vi "4200_strings.vi"() -> ()   [LabVIEW 2013]
panel:
  in  "number 3":dbl
  in  "number 2":dbl
  in  "Number of points":dbl
  in  "SMU2 Output":T1(ring)
  in  "SMU2 Function":enum16{"Sweep", "Step", "Constant"}(ring)
  in  "SMU1 Function":enum16{"Sweep", "Step", "Constant"}(ring)
  in  "SMU1 Output":T1(ring)
  # "SMU2"
  # "SMU1"
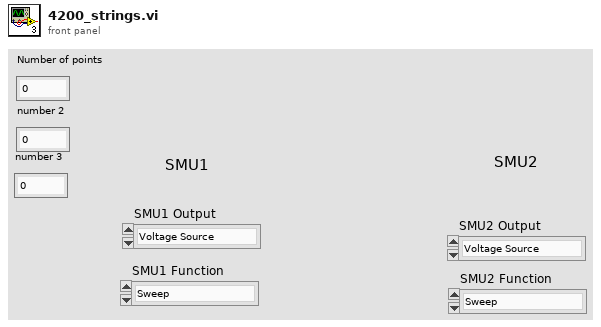
[diagram p1: front panel]
types:
  T1 = enum16{"Voltage Source", "Current Source", "COM"}
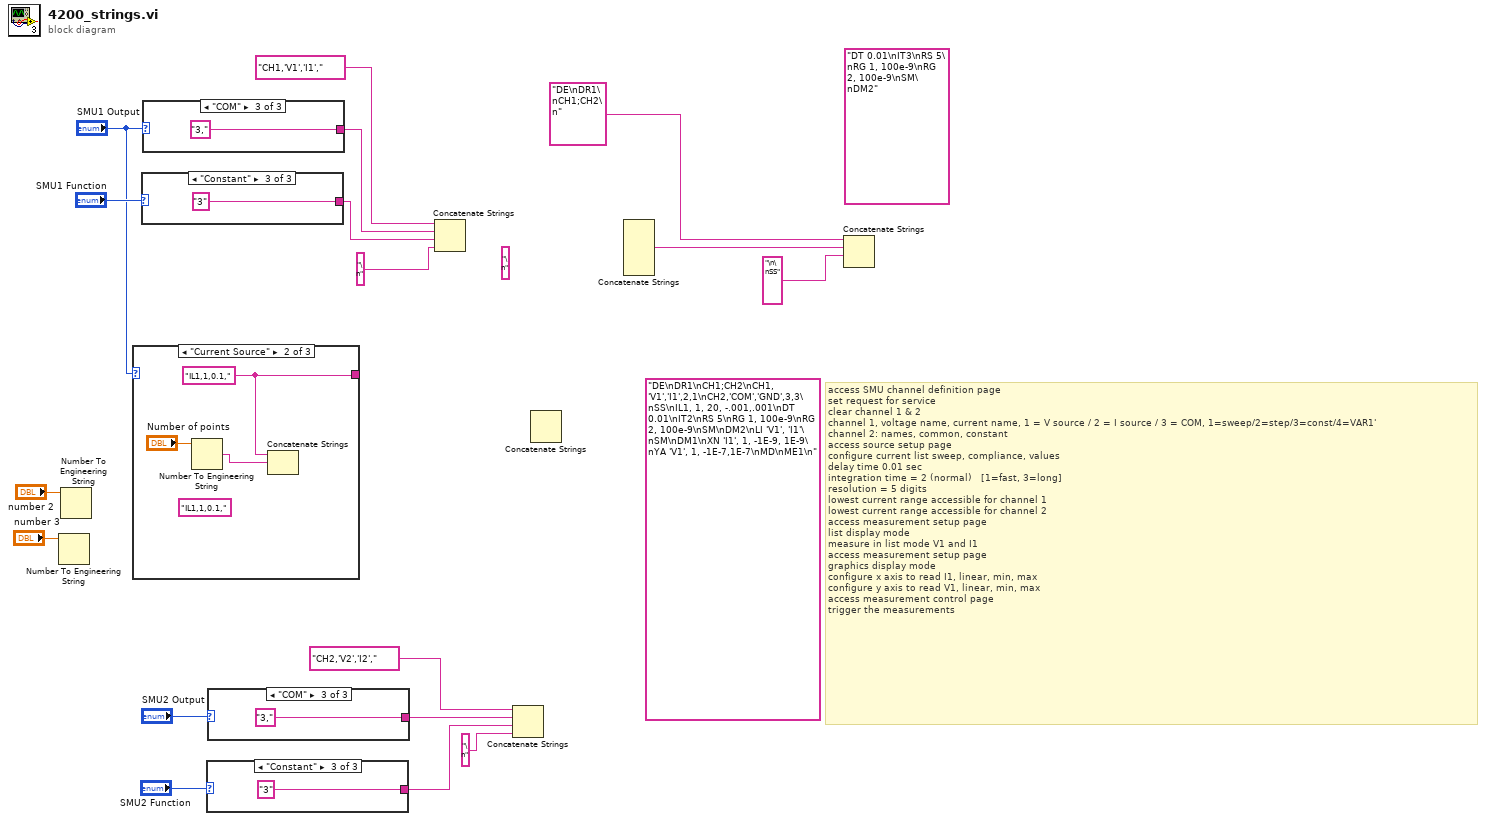
[diagram p0: block diagram]
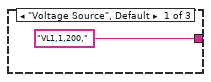
[diagram p2: hidden frame]
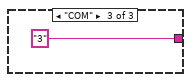
[diagram p3: hidden frame]
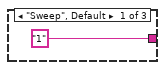
[diagram p4: hidden frame]
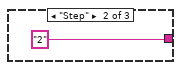
[diagram p5: hidden frame]
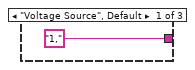
[diagram p6: hidden frame]
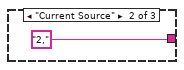
[diagram p7: hidden frame]
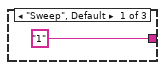
[diagram p8: hidden frame]
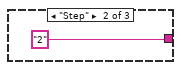
[diagram p9: hidden frame]
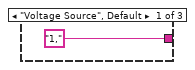
[diagram p10: hidden frame]
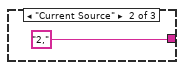
[diagram p11: hidden frame]
diagram:
  (unwired) "DE\nDR1\nCH1;CH2\nCH1, 'V1','I1',2,1\nCH2,'COM','GND',3,3\nSS\nIL1, 1, 20, -.001,.001\nDT 0.01\nIT2\nRS 5\nRG 1, 100e-9\nRG 2, 100e-9\nSM\nDM2\nLI 'V1', 'I1'\nSM\nDM1\nXN 'I1', 1, -1E-9, 1E-9\nYA 'V1', 1, -1E-7,1E-7\nMD\nME1\n" ("write buffer")
  (unwired) "DT 0.01\nIT3\nRS 5\nRG 1, 100e-9\nRG 2, 100e-9\nSM\nDM2" ("string")
  (unwired) "\n" ("string")
  # "access SMU channel definition page\nset request for service\nclear channel 1 & 2\nchannel 1, voltage name, current name, 1 = V source / 2 = I source / 3 = COM, 1=sweep/2=step/3=const/4=VAR1' \nchannel 2: names, common, constant\naccess source setup page\nconfigure current list sweep, compliance, values\ndelay time 0.01 sec\nintegration time = 2 (normal)   [1=fast, 3=long]\nresolution = 5 digits\nlowest current range accessible for channel 1\nlowest current range accessible for channel 2\naccess measurement setup page\nlist display mode\nmeasure in list mode V1 and I1\naccess measurement setup page\ngraphics display mode\nconfigure x axis to read I1, linear, min, max\nconfigure y axis to read V1, linear, min, max\naccess measurement control page\ntrigger the measurements"
  n1 = Number To Engineering String(4:"number 3") -> ()  [unwired: 3 in, 1 out]
  n2 = Number To Engineering String(4:"number 2") -> ()  [unwired: 3 in, 1 out]
  n3 = case shown="\"Current Source\"" "SMU1 Output" {
    tunnel: ["VL1,1,200," ("string") w20 "3" ("string")] -> _
    frame "Voltage Source", Default {
    }
    frame "Current Source" {
      (unwired) "IL1,1,0.1," ("string")
      w20 = "IL1,1,0.1," ("string")
      n4 = Number To Engineering String(4:"Number of points") -> (0:w19:string)  [unwired: 3 in]
      n5 = Concatenate Strings(w20, w19) -> ()  [unwired: 1 in, 1 out]
    }
    frame "COM" {
    }
  }
  n6 = case shown="\"Constant\"" "SMU1 Function" {
    tunnel: ["1" ("string") "2" ("string") "3" ("string")] -> w8
    frame "Sweep", Default {
    }
    frame "Step" {
    }
    frame "Constant" {
    }
  }
  n7 = case shown="\"COM\"" "SMU1 Output" {
    tunnel: ["1," ("string") "2," ("string") "3," ("string")] -> w9
    frame "Voltage Source", Default {
    }
    frame "Current Source" {
    }
    frame "COM" {
    }
  }
  n8 = case shown="\"Constant\"" "SMU2 Function" {
    tunnel: ["1" ("string") "2" ("string") "3" ("string")] -> w5
    frame "Sweep", Default {
    }
    frame "Step" {
    }
    frame "Constant" {
    }
  }
  n9 = case shown="\"COM\"" "SMU2 Output" {
    tunnel: ["1," ("string") "2," ("string") "3," ("string")] -> w6
    frame "Voltage Source", Default {
    }
    frame "Current Source" {
    }
    frame "COM" {
    }
  }
  n10 = Concatenate Strings("CH1,'V1','I1'," ("string"), w9, w8, "\n" ("string")) -> ()  [unwired: 1 out]
  n11 = Concatenate Strings("CH2,'V2','I2'," ("string"), w6, w5, "\n" ("string")) -> ()  [unwired: 1 out]
  n12 = Concatenate Strings() -> ()  [unwired: 4 in, 1 out]
  n13 = Concatenate Strings() -> (w16:string)  [unwired: 7 in]
  n14 = Concatenate Strings("DE\nDR1\nCH1;CH2\n" ("string"), w16, "\n\nSS" ("string")) -> ()  [unwired: 1 in, 1 out]
